vi "Stop Continuous Output.vi"(8 "error in (no error)":errorcluster, 11 "VISA resource name":refnum<visa-resource-name>) -> (0 "error out":errorcluster, 3 "VISA resource name out":refnum<visa-resource-name>)   [LabVIEW 2012, in "MicroStrain 3DM-GXx.lvlib"]
doc: "Stop continuous measurement output."
uses:
  <instrlib>/MicroStrain 3DM-GXx/MicroStrain 3DM-GXx.lvlib
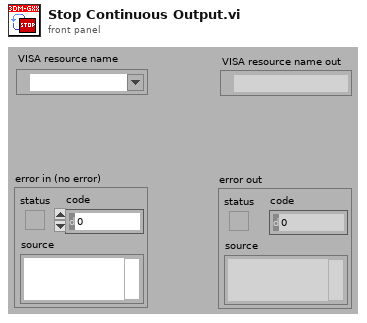
[diagram p1: front panel]
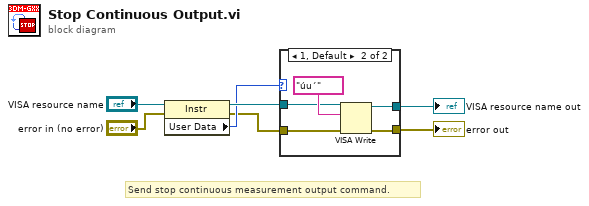
[diagram p0: block diagram]
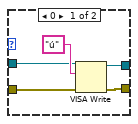
[diagram p2: hidden frame]
diagram:
  # "Send stop continuous measurement output command."
  n1 = property class="Instr"(reference="VISA resource name", error in="error in (no error)") -> (reference out=w3:refnum<visa-resource-name>, error out=w1:errorcluster, "User Data"=w2:u32)
  n2 = case shown="1, Default" w2 {
    tunnel: [w11 w17] -> w7
    tunnel: [w10 w16] -> w6
    tunnel: w3 -> [w8 w14]
    tunnel: w1 -> [w9 w13]
    frame 0 {
      n3 = VISA Write(VISA resource name=w8, write buffer="ú", error in (no error)=w9) -> (VISA resource name out=w11:refnum<visa-resource-name>, error out=w10:errorcluster)  [unwired: 1 out]
    }
    frame 1, Default {
      n4 = VISA Write(VISA resource name=w14, write buffer="úu´", error in (no error)=w13) -> (VISA resource name out=w17:refnum<visa-resource-name>, error out=w16:errorcluster)  [unwired: 1 out]
    }
  }
  "VISA resource name out" <- w7
  "error out" <- w6
